vi "Align To Connector Pane.vi"(6 "Variant in":variant, 7 "Shift Pressed?":bool, 8 "error in (no error)":errorcluster, 10 "QD Combo Box Ref":refnum<vi>, 11 "QD Launch VI Ref":refnum<vi>) -> (0 "error out":errorcluster, 4 "Variant out":variant)   [LabVIEW 2011, in "Align To Connector.lvlib"]
doc: "Aligns controls and indicators to their relative position on the connector pane. \nAlso Resizes and moves the front panel.\n\nIf the block diagram is in focus, this VI will instead size to fit the block diagram.\n\nDefault Shortcut - [A]"
uses:
  Align To Connector Pane Sub VIs/Align To Connector.lvlib
panel:
  # "Do not change the connector pane of this VI.\n\nSee the block diagram for directions on how to use this template."
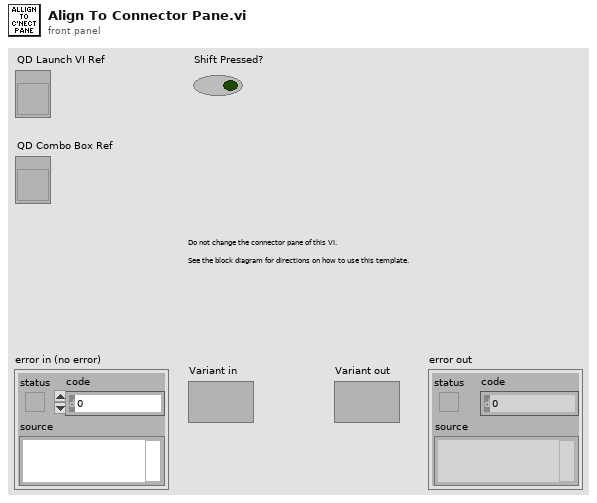
[diagram p1: front panel]
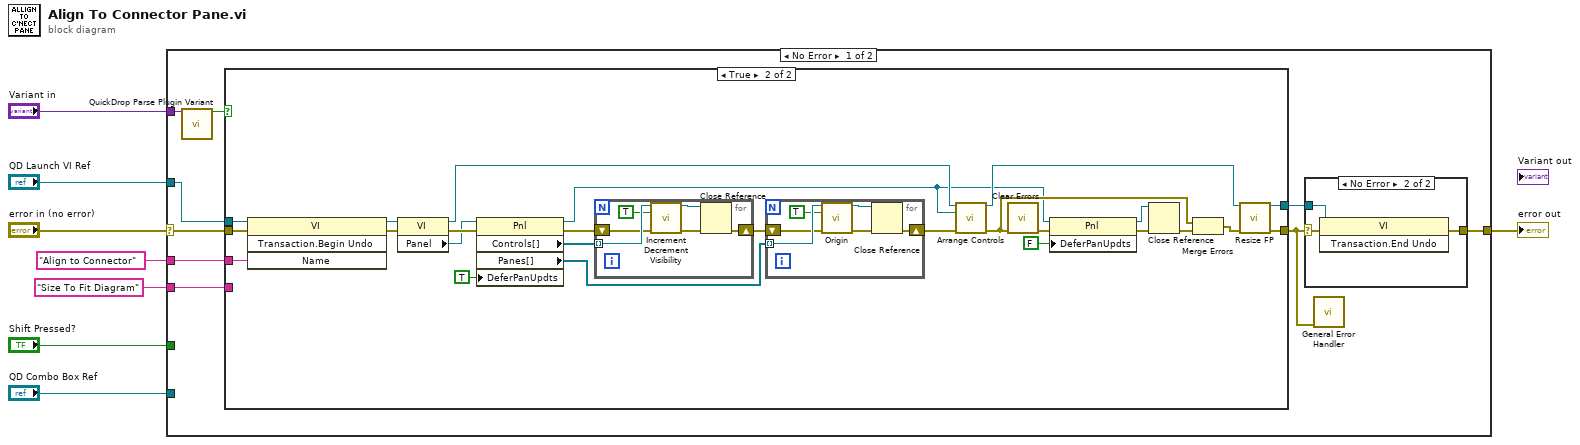
[diagram p0: block diagram]
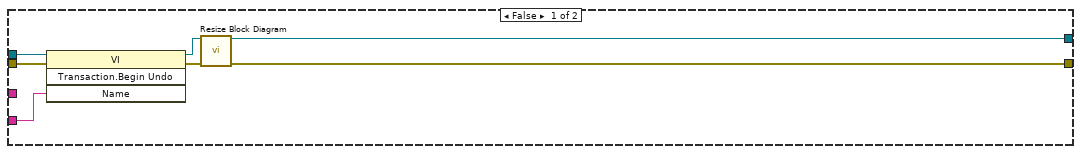
[diagram p2: hidden frame]
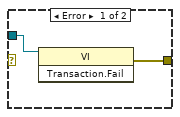
[diagram p3: hidden frame]
diagram:
  n1 = case shown="No Error" "error in (no error)" {
    selector: "error in (no error)" -> [w17 w67]
    tunnel: [w14 w67] -> w7
    tunnel: "QD Launch VI Ref" -> [w16 _]
    tunnel: "Shift Pressed?" -> [_ _]
    tunnel: "QD Combo Box Ref" -> [_ _]
    tunnel: "Variant in" -> [w12 _]
    tunnel: "Align to Connector" ("Undo Name") -> [w15 _]
    tunnel: "Size To Fit Diagram" ("Undo Name") -> [w10 _]
    frame No Error {
      n2 = call <vilib>:"QuickDrop Parse Plugin Variant.vi"("QDKS Variant in"=w12) -> ("QD Launch VI Panel?"=w11:bool)  [unwired: 12 in, 2 out]
      n3 = case shown="True" w11 {
        tunnel: w17 -> [w21 w49]
        tunnel: w16 -> [w22 w48]
        tunnel: w15 -> [_ w47]
        tunnel: [w19 w37] -> w13
        tunnel: [w20 w29] -> w9
        tunnel: w10 -> [w18 _]
        frame False {
          n4 = invoke class="VI" method="Transaction.Begin Undo"(reference=w22, error in=w21, "Name"=w18) -> (reference out=w23:refnum<vi>, error out=w24:errorcluster)  [unwired: 1 in, 2 out]
          n5 = call "Resize Block Diagram.vi"("VI in"=w23, "error in"=w24) -> ("VI out"=w19:refnum<vi>, "error out"=w20:errorcluster)  [unwired: 12 in]
        }
        frame True {
          n6 = invoke class="VI" method="Transaction.Begin Undo"(reference=w48, error in=w49, "Name"=w47) -> (reference out=w46:refnum<vi>, error out=w45:errorcluster)  [unwired: 1 in, 2 out]
          n7 = property class="VI"(reference=w46, error in=w45) -> (reference out=w28:refnum<vi>, error out=w44:errorcluster, "Panel"=w43:refnum<vi>)
          n8 = property class="Pnl"(reference=w43, error in=w44, "DeferPanUpdts"=TRUE ("Defer Panel Updates")) -> (reference out=w27:refnum<vi>, error out=w36:errorcluster, "Controls[]"=w33:refnum<vi>[], "Panes[]"=w34:refnum<vi>[])
          n9 = for {
            tunnel: w33 -> [w52] mode=indexing
            shift-right: [w55] -> w35
            shift-left: w36 -> [w51]
            n10 = call "Increment Decrement Visibility.vi"("Control in"=w52, "make compliant?"=TRUE, "error in"=w51) -> ("Control out"=w54:refnum<vi>, "error out"=w53:errorcluster)  [unwired: 10 in, 1 out]
            n11 = Close Reference(reference=w54, error in (no error)=w53) -> (error out=w55:errorcluster)
          }
          n12 = for {
            tunnel: w34 -> [w58] mode=indexing
            shift-right: [w61] -> w32
            shift-left: w35 -> [w57]
            n13 = call "Origin.vi"("Pane in"=w58, "make compliant?"=TRUE, "error in"=w57) -> ("Pane out"=w60:refnum<vi>, "error out"=w59:errorcluster)  [unwired: 10 in, 1 out]
            n14 = Close Reference(reference=w60, error in (no error)=w59) -> (error out=w61:errorcluster)
          }
          n15 = call "Arrange Controls.vi"("VI in"=w28, "front panel"=w27, "error in"=w32) -> ("VI out"=w38:refnum<vi>, "error out"=w31:errorcluster)  [unwired: 11 in]
          n16 = call <vilib>:"Clear Errors.vi"("error in (no error)"=w31) -> ("error out"=w30:errorcluster)  [unwired: 5 in, 1 out]
          n17 = property class="Pnl"(reference=w27, error in=w30, "DeferPanUpdts"=FALSE ("Defer Panel Updates")) -> (reference out=w40:refnum<vi>, error out=w41:errorcluster)
          n18 = Close Reference(reference=w40, error in (no error)=w41) -> (error out=w26:errorcluster)
          n19 = Merge Errors(w31, w26) -> (w25:errorcluster)
          n20 = call "Resize FP.vi"("VI in"=w38, "error in"=w25) -> ("VI out"=w37:refnum<vi>, "error out"=w29:errorcluster)  [unwired: 12 in]
        }
      }
      n21 = case shown="No Error" w9 {
        selector: w9 -> [_ w64]
        tunnel: w13 -> [w62 w65]
        tunnel: [w63 w66] -> w14
        frame Error {
          n22 = invoke class="VI" method="Transaction.Fail"(reference=w62) -> (error out=w63:errorcluster)  [unwired: 2 in, 2 out]
        }
        frame No Error {
          n23 = invoke class="VI" method="Transaction.End Undo"(reference=w65, error in=w64) -> (error out=w66:errorcluster)  [unwired: 1 in, 2 out]
        }
      }
      n24 = call <vilib>:"General Error Handler.vi"("error in (no error)"=w9) -> ()  [unwired: 10 in, 5 out]
    }
    frame Error {
    }
  }
  "error out" <- w7
